vi "getImageRefGray.vi"(8 "error in (no error)":errorcluster, 11 "camera in":refnum<class "camera.lvclass">) -> (0 "error out":errorcluster, 2 "Image":T1, 3 "camera out":refnum<class "camera.lvclass">)   [LabVIEW 2017, in "camera.lvclass"]
uses:
  camera.lvclass
  <vilib>/vision/Image Controls.llb/IMAQ Image.ctl
  camera.lvclass/camera.ctl
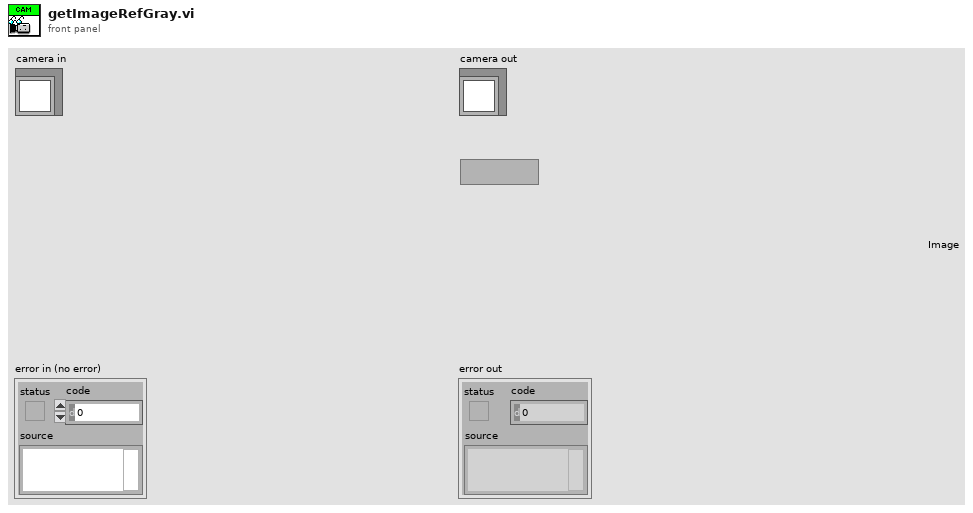
[diagram p1: front panel]
types:
  T1 = typedef "IMAQ Image.ctl" = refnum<image>
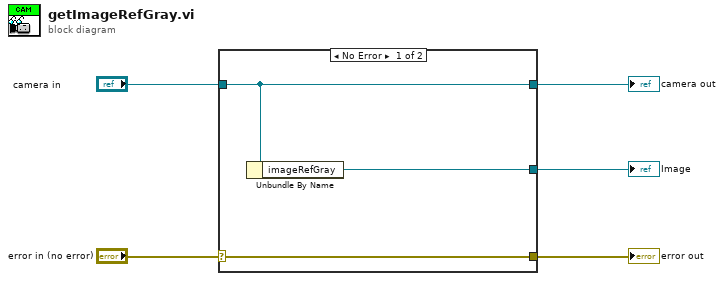
[diagram p0: block diagram]
diagram:
  n1 = case shown="No Error" "error in (no error)" {
    selector: "error in (no error)" -> [w8 w9]
    tunnel: [w8 w9] -> w4
    tunnel: [w7 w10] -> w2
    tunnel: "camera in" -> [w7 w10]
    tunnel: [w6 _] -> w1
    frame No Error {
      n2 = Unbundle By Name(w7) -> ("imageRefGray"=w6:T1)
    }
    frame Error {
    }
  }
  "error out" <- w4
  "camera out" <- w2
  "Image" <- w1
